vi "ziExample-ListDevices.vi"() -> ()   [LabVIEW 2009]
doc: "Control a Zurich instrument device via the LabOne Labview API. \nRequirements: Zurich Instruments MFLI, HF2 or UHFLI \nThis is an example for the Zurich Instruments LabOne LabVIEW API. This example lists all available instruments and displays some information on them.\n\n© Zurich Instruments AG, www.zhinst.com"
uses:
  <instrlib>/Zurich Instruments LabOne/Zurich Instruments LabOne.lvlib
panel:
  in  "port":u16(ring)=8005 caption="Port" items=["HF2 Series (8005)"=8005, "UHF Series (8004)"=8004]
  out "Selected Device":string
  out "Devices":cluster{"Device":string, "Demods":i32}[](array[cluster])
  out "Error Out":errorcluster
  out "Nodes":string[](array[string])
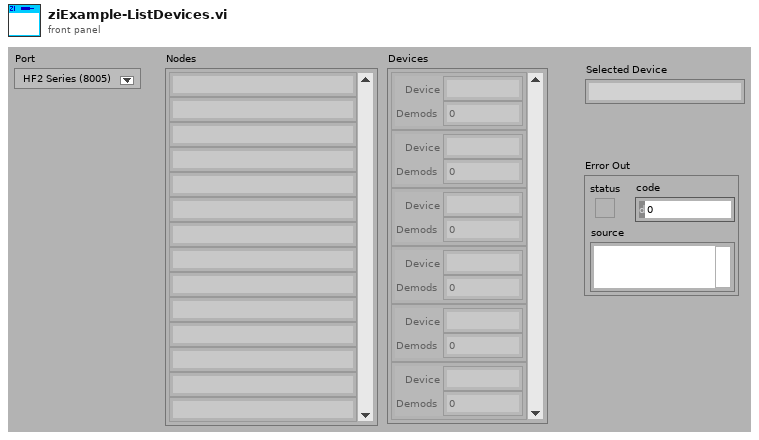
[diagram p1: front panel]
types:
  T1 = typedef "Zurich Instruments LabOne.lvlib/ziTypeHandle.ctl" = cluster{"handleValid":bool, "Conn":u64, "Path Prefix":string, "Handle":u64, "Connected":bool, "Clockbase(s)":dbl}
  T2 = cluster{"Recursive":bool, "Absolut":bool, "Leafs Only":bool, "Settings Only":bool}
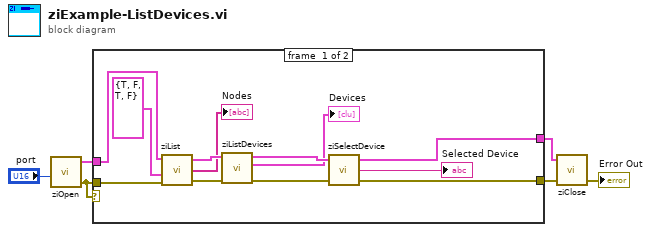
[diagram p0: block diagram]
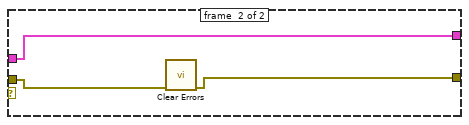
[diagram p2: hidden frame]
diagram:
  n1 = call <instrlib>:"ziOpen.vi"("Port obsolete (auto)"="port") -> ("Error Out"=w1:errorcluster, "HandleOut"=w6:T1)  [unwired: 3 in, 1 out]
  n2 = case shown="Error" w1 {
    tunnel: w6 -> [w18 w21]
    tunnel: [w12 w19] -> w4
    tunnel: [w11 w21] -> w3
    tunnel: w1 -> [w7 w20]
    frame #0 {
      n3 = call <instrlib>:"ziList.vi"("Error In"=w7, "Flags (None)"=T2 {"Recursive"=TRUE, "Absolut"=FALSE, "Leafs Only"=TRUE, "Settings Only"=FALSE}, "Handle In"=w18) -> ("Error Out"=w8:errorcluster, "Nodes"=→"Nodes":string[], "Handle Out"=w17:T1)  [unwired: 1 in]
      n4 = call <instrlib>:"ziListDevices.vi"("Error In"=w8, "Handle In"=w17) -> ("Error Out"=w16:errorcluster, "Devices"=→"Devices":cluster{"Nodes":string, i32}[], "Handle Out"=w15:T1)  [unwired: 3 in]
      n5 = call <instrlib>:"ziSelectDevice.vi"("Error In"=w16, "Handle In"=w15) -> ("Error Out"=w12:errorcluster, "Selected Device"=→"Selected Device":string, "Handle Out"=w11:T1)  [unwired: 1 in]
    }
    frame #1 {
      n6 = call <vilib>:"Clear Errors.vi"("error in (no error)"=w20) -> ("error out"=w19:errorcluster)  [unwired: 6 in]
    }
  }
  n7 = call <instrlib>:"ziClose.vi"("Error In"=w4, "Handle In"=w3) -> ("Error Out"=→"Error Out":errorcluster)  [unwired: 2 in, 1 out]
